vi "SUB_VI_scrittura_messaggio_client_T_Oss_array.vi"(8 "Errore in ingresso":errorcluster, 9 "Freq.Campionamento":dbl, 10 "T.Osservazione":dbl, 11 "TCP Network Connection in":refnum<k5>) -> (0 "Errore in uscita":errorcluster, 3 "TCP Network Connection out":refnum<k5>)   [LabVIEW 2023]
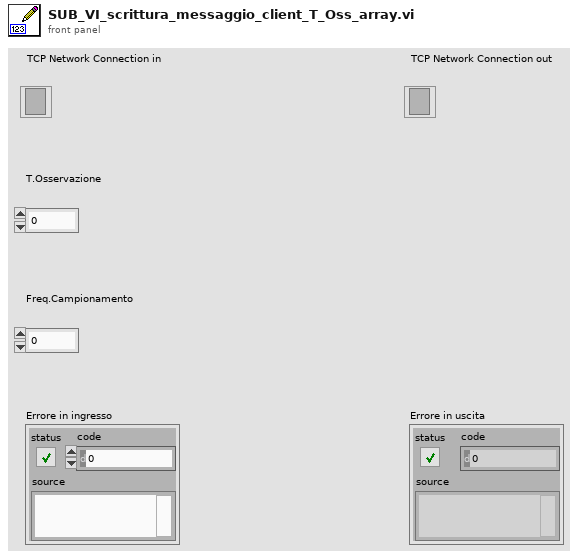
[diagram p1: front panel]
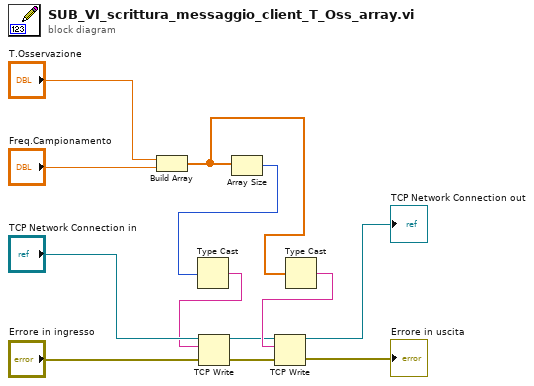
[diagram p0: block diagram]
diagram:
  n1 = Build Array("T.Osservazione", "Freq.Campionamento") -> (w7:dbl[])
  n2 = Array Size(array=w7) -> (size(s)=w6:i32)
  n3 = Type Cast(x=w6) -> (*(type *) &x=w1:string)  [unwired: 1 in]
  n4 = TCP Write(connection ID="TCP Network Connection in", data in=w1, error in (no error)="Errore in ingresso") -> (connection ID out=w2:refnum<k5>, error out=w5:errorcluster)  [unwired: 1 in, 1 out]
  n5 = Type Cast(x=w7) -> (*(type *) &x=w8:string)  [unwired: 1 in]
  n6 = TCP Write(connection ID=w2, data in=w8, error in (no error)=w5) -> (connection ID out=→"TCP Network Connection out":refnum<k5>, error out=→"Errore in uscita":errorcluster)  [unwired: 1 in, 1 out]
